vi "get_output_status.vi"(8 "error in":errorcluster, 11 "VISA resource name":refnum<visa-resource-name>="COM1") -> (0 "error out":errorcluster, 3 "Response":string)   [LabVIEW 2020]
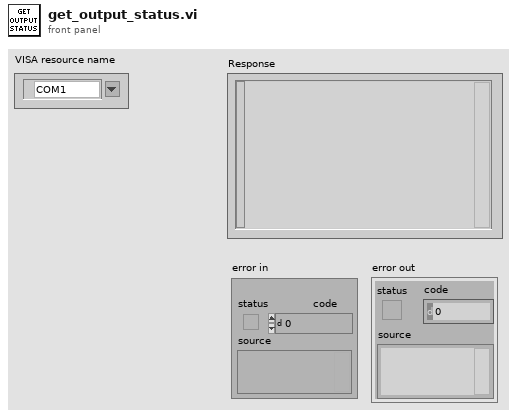
[diagram p1: front panel]
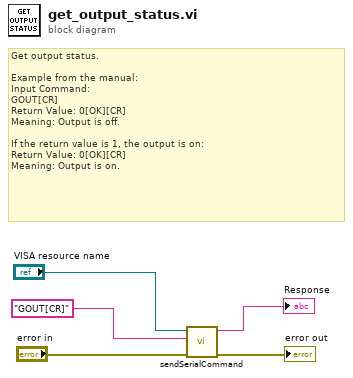
[diagram p0: block diagram]
diagram:
  # "Get output status.\n\nExample from the manual:\nInput Command:\nGOUT[CR]\nReturn Value: 0[OK][CR]\nMeaning: Output is off.\n\nIf the return value is 1, the output is on:\nReturn Value: 0[OK][CR]\nMeaning: Output is on."
  n1 = call "sendSerialCommand.vi"("error in (no error)"="error in", "Command"="GOUT[CR]", "VISA resource name"="VISA resource name") -> ("error out"=→"error out":errorcluster, "Response"=→"Response":string)  [unwired: 7 in]
